vi "GETmap.vi"(7 "LabVIEW Web Service Request":refnum<class "Web Request.lvclass">) -> (3 "LabVIEW Web Service Request out":refnum<class "Web Request.lvclass">)   [LabVIEW 2014]
uses:
  <vilib>/wsapi/Web Request.lvclass
  Libraries/Map Data Folder/Map Data.lvlib
panel:
  # "Use the Web Service Request input terminal to call the VIs on the Web Services palette. Do not remove it from the connector pane unless you don't need access to the palette."
  # "Each additional control wired to the connector pane will be available as an input in the URL. To include an indicator in terminal-mode output (the default setting), it must also be wired to the connector pane."
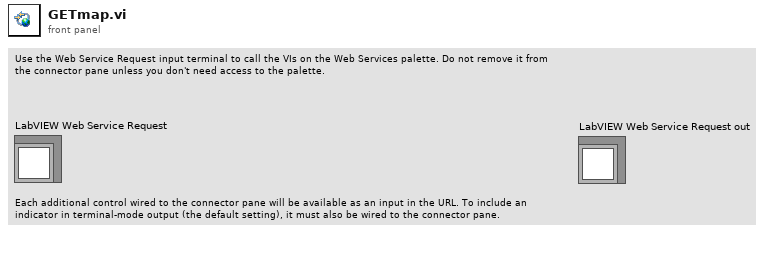
[diagram p1: front panel]
types:
  T1 = typedef "Map Data.lvlib/All-Lines.ctl" = T2[]
  T2 = typedef "Map Data.lvlib/LineCluster.ctl" = cluster{"Line name":string, "Line array":cluster{"X":dbl, "Y":dbl, "Z":dbl}[], "Line connections":T3[]}
  T3 = typedef "LineConnection.ctl" = cluster{"Index":i32, "Switch Pos":cluster{"X":dbl, "Y":dbl, "Z":dbl}, "Switch operational":bool, "Switch State":bool, "Connection Index":i32, "Connection Pos":cluster{"X":dbl, "Y":dbl, "Z":dbl}, "LinePos Index":i32, "ConnectPos Index":i32, "Same direction?":bool, "Manual Overide":bool, "Manual State":bool}
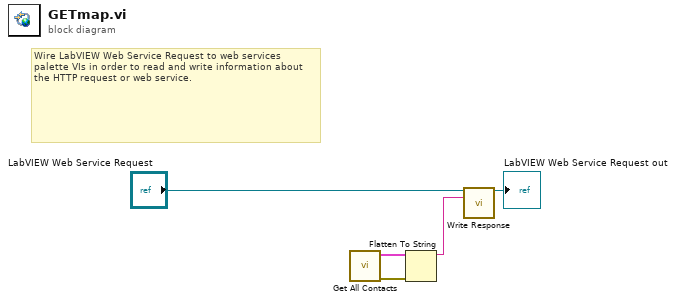
[diagram p0: block diagram]
diagram:
  # "Wire LabVIEW Web Service Request to web services palette VIs in order to read and write information about the HTTP request or web service."
  n1 = call "Get All Contacts.vi"() -> ("error out"=w4:errorcluster, "All Lines out"=w5:T1)  [unwired: 9 in, 1 out]
  n2 = Flatten To String(anything=w5, error in (no error)=w4) -> (data string=w2:string)  [unwired: 2 in, 2 out]
  n3 = call <vilib>:"Write Response.vi"("LabVIEW Web Service Request"="LabVIEW Web Service Request", "response string"=w2) -> ("LabVIEW Web Service Request out"=→"LabVIEW Web Service Request out":refnum<class "Web Request.lvclass">)  [unwired: 12 in, 1 out]
